vi "Generate File List.vi"(8 "error in (no error)":errorcluster, 10 "filename":string, 11 "Save Path":path=path "E:/Jiarui/1217test") -> (0 "error out":errorcluster)   [LabVIEW 2017]
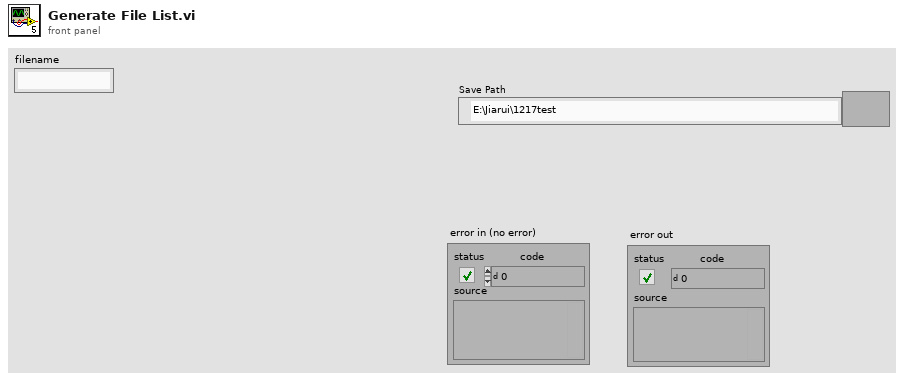
[diagram p1: front panel]
types:
  T1 = enum16{"open", "replace", "create", "open or create", "replace or create", "replace or create with confirmation"}
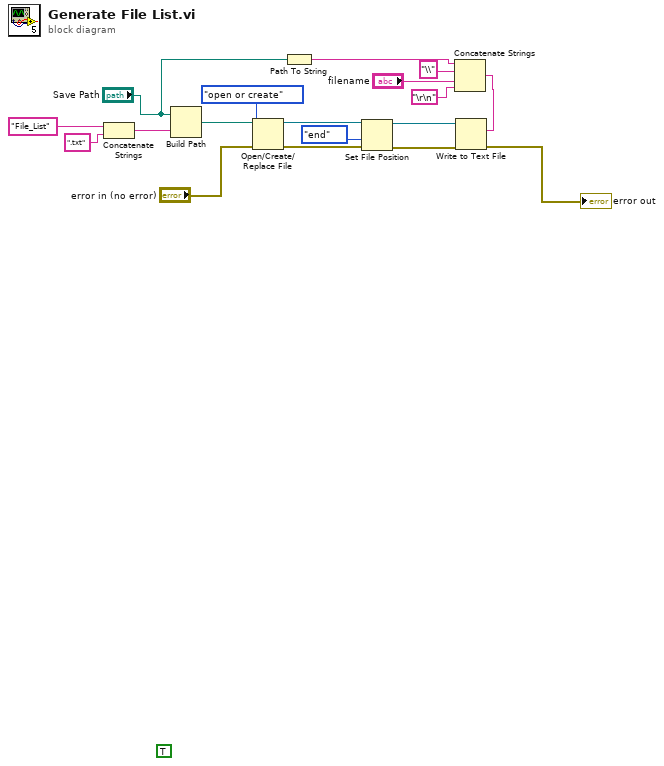
[diagram p0: block diagram]
diagram:
  (unwired) TRUE
  n1 = Concatenate Strings("File_List" ("string"), ".txt" ("string")) -> (w16:string)
  n2 = Build Path(base path="Save Path", name or relative path=w16) -> (appended path=w12:path)
  n3 = Open/Create/Replace File(file path (use dialog)=w12, error in="error in (no error)", operation (0:open)=T1."open or create") -> (refnum out=w5:refnum<file>, error out=w7:errorcluster)  [unwired: 3 in, 1 out]
  n4 = Path To String(path="Save Path") -> (string=w2:string)
  n5 = Set File Position(refnum=w5, from (0:start)=enum16{"start", "end", "current"}."end", error in=w7) -> (refnum out=w4:refnum<file>, error out=w6:errorcluster)  [unwired: 1 in]
  n6 = Concatenate Strings(w2, "\\" ("string"), "filename", "\r\n" ("string")) -> (w10:string)
  n7 = Write to Text File(file (use dialog)=w4, text=w10, error in=w6) -> (error out=→"error out":errorcluster)  [unwired: 1 in, 2 out]
